vi "UHR-Fleezers Control (host) - 16.2.2v2.vi"() -> ()   [LabVIEW 2014] (continued)
        n2296 = Negate(x=w3289) -> (-x=w3285:dbl)
        n2297 = local write "Scan Range (nm)"(w3285) -> ()
        n2298 = Divide(x=w3311, y=w3339) -> (x/y=w3295:dbl)
        "Scan Increment (MHz)" <- w3295
        n2299 = call "IR AOM freq to word.vi"("Frequency In (MHz)"=w3295) -> ("Frequency Word Out (double)"=w3294:dbl)
        n2300 = Divide(x="Step Size (nm)", y="Scan Speed (nm/s)") -> (x/y=w3282:dbl)
        n2301 = To Quad Integer(1:w3294) -> ()  [unwired: 1 out]
        n2302 = local read "Number Interlace Sets"() -> (w3266:u8)
        n2303 = local read "AI Count (ticks)"() -> (w3267:u16)
        n2304 = local read "Total Counts (ticks)"() -> (w3265:u16)
        n2305 = local read "# Samples/trap"() -> (w3297:u32)
        n2306 = Multiply(x=w3267, y=w3266) -> (x*y=w3264:u16)
        n2307 = Divide(x=w3265, y=w3264) -> (x/y=w3263:dbl)
        n2308 = Select(t=w3298, s="Scan BD", f=w3304) -> (s? t:f=w3336:dbl)
        "Initial freq. (MHz)" <- w3336
        n2309 = Add(x=w3311, y=w3336) -> (x+y=→"Final freq. (MHz)":dbl)
        n2310 = Divide(x=w3265, y=40000000.0) -> (x/y=w3281:dbl)
        n2311 = Divide(x=w3282, y=w3281) -> (x/y=w3280:dbl)
        n2312 = To Unsigned Quad Integer(1:w3280) -> (0:w3255:u64)
        n2313 = Quotient & Remainder(x=w3255, y=u64 2) -> (x-y*floor(x/y)=w3259:u64)  [unwired: 1 out]
        n2314 = Equal?(x=w3259, y=u64 0) -> (x = y?=w3257:bool)
        n2315 = Decrement(x=w3255) -> (x-1=w3256:u64)
        n2316 = Select(t=w3255, s=w3257, f=w3256) -> (s? t:f=w3254:u64)
        "Cycles/step (AOD)" <- w3254
        n2317 = xnode "Read/Write Control"("FPGA VI Reference In"=w3253, "Scan steps"=w3286, "Number of scans"="Number of F/B Scans (AOD)", "Cycles per step"=w3254, "Scan freq.  increment"=w3292, "Scan BD"="Scan BD") -> ("error out"=w3345:errorcluster)  [unwired: 1 in, 1 out]
        n2318 = Multiply(x=w3286, y=w3254) -> (x*y=w3340:u64)
        n2319 = Multiply(x=w3340, y=u64 2) -> (x*y=w3262:u64)
        n2320 = Multiply(x=w3263, y=w3262) -> (x*y=w3261:dbl)
        "Data points/scan (f/b)" <- w3261
        n2321 = Multiply(x=w3261, y="Number of F/B Scans (AOD)") -> (x*y=w3343:dbl)
        "Data points/scans" <- w3343
        n2322 = Divide(x=w3343, y=w3297) -> (x/y=→"N sets should be saved":dbl)
        n2323 = Multiply(x=w3340, y=w3281) -> (x*y=w3279:dbl)
        "Time/Scan (s) (AOD)" <- w3279
        n2324 = Select(t=w3311, s="Scan BD", f=0.0) -> (s? t:f=w3337:dbl)
        n2325 = Select(t=0.0, s="Scan BD", f=w3311) -> (s? t:f=w3333:dbl)
        n2326 = local read "BD 2 Frequency 2 (MHz)"() -> (w3329:dbl)
        n2327 = local read "BD 1 Frequency 2 (MHz)"() -> (w3332:dbl)
        n2328 = Add(x=w3333, y=w3304) -> (x+y=w3330:dbl)
        n2329 = Add(x=w3298, y=w3337) -> (x+y=w3331:dbl)
        n2330 = Multiply(x=w3279, y=2.0) -> (x*y=w3278:dbl)
        n2331 = Multiply(x=w3278, y="Number of F/B Scans (AOD)") -> (x*y=w3275:dbl)
        n2332 = Divide(x=w3275, y=60.0) -> (x/y=→"Time to Finish All (min)":dbl)
        n2333 = Add(x="Trap 2 Bead Size (nm)", y="Trap 1 Bead Size (nm)") -> (x+y=w3319:dbl)
        n2334 = Divide(x=w3319, y=2.0) -> (x/y=w3313:dbl)
        n2335 = local read "Initial delta (MHz)"() -> (w3316:dbl)
        n2336 = Subtract(x=w3330, y=w3329) -> (x-y=w3327:dbl)
        n2337 = Subtract(x=w3331, y=w3332) -> (x-y=w3328:dbl)
        n2338 = Square(x=w3327) -> (x^2=w3326:dbl)
        n2339 = Square(x=w3328) -> (x^2=w3325:dbl)
        n2340 = Add(x=w3325, y=w3326) -> (x+y=w3324:dbl)
        n2341 = Square Root(x=w3324) -> (sqrt(x)=w3323:dbl)
        "Final delta (MHz)" <- w3323
        n2342 = Multiply(x=w3315, y=w3323) -> (x*y=w3322:dbl)
        n2343 = Multiply(x=w3316, y=w3315) -> (x*y=w3314:dbl)
        n2344 = Subtract(x=w3314, y=w3313) -> (x-y=→"Initial sep (nm)":dbl)
        n2345 = Subtract(x=w3322, y=w3313) -> (x-y=→"Final sep (nm)":dbl)
      }
      event "Swap F1 and F2", "RF amplitude switch delay": Value Change {
        n2346 = event-data() -> ()  [unwired: 7 out]
        n2347 = local read "RF amplitude switch delay"() -> (w3347:u16)
        n2348 = local read "Swap F1 and F2"() -> (w3348:bool)
        n2349 = xnode "Read/Write Control"("FPGA VI Reference In"=w3346, "Swap F1 and F2"=w3348, "Amp switch delay"=w3347) -> ("error out"=w3349:errorcluster)  [unwired: 1 in, 1 out]
      }
      event "Scan steps (MCL)", "Number of scans (MCL)", "Scan Range (V)\n(of steps)", "2D or 1D Scan", "N APD Samp/step", "Fast Scan Dir", "Continuous MCL Scanning", "Scan lines (y)": Value Change {
        w3353 = 32767.0 ("y")
        n2350 = event-data() -> ()  [unwired: 7 out]
        n2351 = Select(t="Scan lines (y)", s="2D or 1D Scan", f="Number of scans (MCL)") -> (s? t:f=w3358:u64)
        n2352 = local read "Host fluorescence integration time (s)"() -> (w3350:dbl)
        n2353 = Decrement(x="Scan steps (MCL)") -> (x-1=w3373:u64)
        n2354 = Divide(x="Scan Range (V)\n(of steps)", y=w3373) -> (x/y=w3372:dbl)
        "Desired Scan Incr (V)" <- w3372
        n2355 = Multiply(x=w3372, y=w3353) -> (x*y=w3381:dbl)
        n2356 = Divide(x=w3381, y=10.0) -> (x/y=w3371:dbl)
        "Desired incr (int)" <- w3371
        n2357 = local read "Update Count (MCL)"() -> (w3377:u32)
        n2358 = Round Toward -Infinity(1:w3371) -> (0:w3380:dbl)
        n2359 = To Word Integer(number=w3380) -> (16bit integer=w3356:i16)
        "Actual Incr. int (MCL)" <- w3356
        n2360 = Multiply(x=w3350, y=40000000.0) -> (x*y=w3378:dbl)
        n2361 = Divide(x=w3378, y=w3377) -> (x/y=w3376:dbl)
        n2362 = Multiply(x=i16 10, y=w3356) -> (x*y=w3354:i16)
        n2363 = Multiply(x="N APD Samp/step", y=w3376) -> (x*y=w3375:dbl)
        "Cycles/step (MCL)" <- w3375
        n2364 = Divide(x=w3354, y=w3353) -> (x/y=→"Actual MCL Inc (V)":dbl)
        n2365 = Multiply(x="N APD Samp/step", y="Scan steps (MCL)") -> (x*y=w3367:dbl)
        n2366 = local read "APD Samples/FIFO Acq."() -> (w3365:dbl)
        n2367 = Multiply(x=w3367, y=u64 2) -> (x*y=w3366:dbl)
        "Data points/scan (f+b)" <- w3366
        n2368 = Multiply(x=w3366, y=w3358) -> (x*y=w3384:dbl)
        "Data points/scans (MCL)" <- w3384
        n2369 = Multiply(x=w3350, y=w3366) -> (x*y=w3359:dbl)
        "Time/f+b scan (s) (MCL)" <- w3359
        n2370 = Divide(x=w3384, y=w3365) -> (x/y=→"N sets should be saved (MCL)":dbl)
        n2371 = Multiply(x=w3359, y=w3358) -> (x*y=→"Total Time (s)":dbl)
        n2372 = Not(x="Fast Scan Dir") -> (.not. x?=w3363:bool)
        n2373 = xnode "Read/Write Control"("FPGA VI Reference In"=w3351, "Scan steps (MCL)"="Scan steps (MCL)", "Number of scans (MCL)"=w3358, "Cycles per step (MCL)"=w3375, "Scan freq.  increment (MCL)"=w3356, "1D or 2D Scan?"="2D or 1D Scan", "MCL Scan Axis"=w3363, "Cont. Scan (MCL)"="Continuous MCL Scanning") -> ("error out"=w3386:errorcluster)  [unwired: 1 in, 1 out]
      }
      event "Read Cal": Value Change {
        w3398 = 1000.0 ("y")
        n2374 = event-data() -> ()  [unwired: 7 out]
        n2375 = local read "Save file name"() -> (w3417:path)
        n2376 = local write "Read Cal"(FALSE ("Read Cal")) -> ()
        n2377 = Strip Path(path=w3417) -> (stripped path=w3416:path)  [unwired: 1 out]
        n2378 = Path To String(path=w3416) -> (string=w3415:string)
        n2379 = Concatenate Strings(w3415, "\\current.cal" ("string")) -> (w3413:string)
        n2380 = String To Path(string=w3413) -> (path=w3412:path)
        n2381 = Open/Create/Replace File(file path (use dialog)=w3412, operation (0:open)=T35."open", access (0:read/write)=enum16{"read/write", "read-only", "write-only"}."read-only") -> (refnum out=w3420:refnum<file>, error out=w3406:errorcluster)  [unwired: 1 in, 3 out]
        n2382 = Deny Access(4:w3406, 7:w3420) -> (0:w3405:errorcluster, 3:w3411:refnum<file>)  [unwired: 1 out]
        n2383 = Read from Binary File(5:0.0, 8:w3405, 9:T34."big-endian, network order" ("byte order (0:big-endian, network order)"), 10:-1 ("count (1)"), 11:w3411) -> (0:w3404:errorcluster, 2:w3402:dbl[], 3:w3407:refnum<file>)  [unwired: 2 out]
        n2384 = Array To Cluster(array=w3402) -> (cluster=w3401:T39)
        n2385 = Unbundle(w3401) -> ("[0]"=w3395:dbl, "[1]"=w3389:dbl, "[2]"=w3393:dbl, "[3]"=w3387:dbl, "[4]"=w3400:dbl, "[5]"=w3399:dbl)
        n2386 = Close File(refnum=w3407, error in=w3404) -> (error out=→"Read cal error":errorcluster)  [unwired: 1 out]
        n2387 = Multiply(x=w3400, y=w3398) -> (x*y=w3394:dbl)
        n2388 = Multiply(x=w3399, y=w3398) -> (x*y=w3388:dbl)
        n2389 = Bundle By Name(cluster="T1 calibration", "T1 alpha_x (nm/V)"=w3395, "T1 offset_x (mV)"=w3394, "T1 kappa_x (pN/nm)"=w3393) -> (w3392:T6)
        n2390 = Bundle By Name(cluster="T2 calibration", "T2 alpha_x (nm/V)"=w3389, "T2 offset_x (mV)"=w3388, "T2 kappa_x (pN/nm)"=w3387) -> (w3390:T5)
        n2391 = local write "T1 calibration"(w3392) -> ()
        n2392 = local write "T2 calibration"(w3390) -> ()
      }
      event "Abort MCL Scan": Value Change {
        n2393 = event-data() -> ()  [unwired: 7 out]
        n2394 = local write "MCL Scanning"(FALSE ("MCL Scanning")) -> ()
        n2395 = xnode "Read/Write Control"("FPGA VI Reference In"=w3421, "Abort scan (MCL)"="Abort MCL Scan") -> ("error out"=w3424:errorcluster)  [unwired: 1 in, 1 out]
      }
      event "Update Count (MCL)": Value Change {
        n2396 = event-data() -> ()  [unwired: 7 out]
        n2397 = xnode "Read/Write Control"("FPGA VI Reference In"=w3425, "MCL count"="Update Count (MCL)") -> ("error out"=w3427:errorcluster)  [unwired: 1 in, 1 out]
      }
      event "+ phase (MCL)", "- phase (MCL)": Value Change {
        n2398 = event-data() -> ()  [unwired: 7 out]
        n2399 = Or(x="- phase (MCL)", y="+ phase (MCL)") -> (x .or. y?=w3431:bool)
        n2400 = Negate(x="Phase adjust (MCL)") -> (-x=w3437:i16)
        n2401 = Select(t=w3437, s="+ phase (MCL)", f="Phase adjust (MCL)") -> (s? t:f=w3435:i16)
        n2402 = xnode "Read/Write Control"("FPGA VI Reference In"=w3428, "Phase count adjustment (MCL)"=w3435) -> ("FPGA VI Reference Out"=w3432:T25, "error out"=w3433:errorcluster)  [unwired: 1 in]
        n2403 = xnode "Read/Write Control"("FPGA VI Reference In"=w3432, "error in"=w3433, "+ phase (MCL)"=w3431) -> ("error out"=w3430:errorcluster)  [unwired: 1 out]
      }
      event "Abort AOD Scan": Value Change {
        n2404 = event-data() -> ()  [unwired: 7 out]
        n2405 = xnode "Read/Write Control"("FPGA VI Reference In"=w3438, "Abort scan"="Abort AOD Scan") -> ("error out"=w3440:errorcluster)  [unwired: 1 in, 1 out]
      }
      event "Continuous AOD Scanning": Value Change {
        n2406 = event-data() -> ()  [unwired: 7 out]
        n2407 = xnode "Read/Write Control"("FPGA VI Reference In"=w3441, "Cont. Scan"="Continuous AOD Scanning") -> ("error out"=w3443:errorcluster)  [unwired: 1 in, 1 out]
      }
      event "Index": Value Change {
        n2408 = event-data() -> ()  [unwired: 7 out]
        n2409 = call "Create new save file.vi"("Insert"="", "Ext"=".dat" ("string"), "Index In"="Index") -> ("Path Out"=→"Save file name":path, "Index Out"=w3444:dbl)
        "Save index" <- w3444
        n2410 = local write "Index"(w3444) -> ()
      }
      event "AO1", "AO2": Value Change {
        w3458 = 10.0 ("y")
        w3457 = 32767.0 ("y")
        n2411 = event-data() -> ()  [unwired: 7 out]
        n2412 = local read "AO2"() -> (w3456:dbl)
        n2413 = local read "AO1"() -> (w3453:dbl)
        n2414 = Multiply(x=w3453, y=w3457) -> (x*y=w3452:dbl)
        n2415 = Multiply(x=w3456, y=w3457) -> (x*y=w3455:dbl)
        n2416 = Divide(x=w3452, y=w3458) -> (x/y=w3451:dbl)
        n2417 = Divide(x=w3455, y=w3458) -> (x/y=w3454:dbl)
        n2418 = To Word Integer(number=w3451) -> (16bit integer=w3459:i16)
        n2419 = To Word Integer(number=w3454) -> (16bit integer=w3460:i16)
        n2420 = xnode "Read/Write Control"("FPGA VI Reference In"=w3449, "AO1"=w3459, "AO2"=w3460) -> ("error out"=w3450:errorcluster)  [unwired: 1 in, 1 out]
      }
      event "Inject Pump 1": Value Change {
        n2421 = event-data() -> ()  [unwired: 7 out]
        n2422 = local read "Use Harvard pumps\nfor beads (else Chemyx)"() -> (w3462:bool)
        n2423 = case shown="True" w3462 {
          tunnel: "Inject Pump 1" -> [w3466 w3507]
          tunnel: w3461 -> [_ w3508]
          frame False {
            n2424 = local read "Pump write delay (ms)"() -> (w3465:dbl)
            n2425 = local read "Chemyx Syringe Pump Serial Port"() -> (w3464:refnum<visa-resource-name>)
            n2426 = case shown="True" w3466 {
              tunnel: w3465 -> [w3472 w3486]
              tunnel: w3464 -> [w3469 w3485]
              frame False {
                n2427 = flat-sequence {
                  tunnel: w3469 -> [w3473]
                  tunnel: [w3473] -> w3470
                  tunnel: w3472 -> [_]
                  tunnel: [w3476] -> w3471
                  tunnel: w3470 -> [w3476]
                  tunnel: w3471 -> [w3477]
                  tunnel: [w3477] -> w3467
                  tunnel: [w3479] -> w3468
                  tunnel: w3467 -> [w3479]
                  tunnel: w3468 -> [w3481]
                  frame #0 {
                    n2428 = call "Write to pump.vi"("string"="enter pump1", "VISA resource name"=w3473) -> ()  [unwired: 1 out]
                  }
                  frame #1 {
                    n2429 = Wait (ms)(milliseconds to wait="Pump pause delay (ms)") -> ()  [unwired: 1 out]
                  }
                  frame #2 {
                    n2430 = call "Write to pump.vi"("string"="stop", "VISA resource name"=w3477) -> ()  [unwired: 1 out]
                  }
                  frame #3 {
                    n2431 = Wait (ms)(milliseconds to wait=u32 500) -> ()  [unwired: 1 out]
                  }
                  frame #4 {
                    n2432 = call "Write to pump.vi"("string"="stop", "VISA resource name"=w3481) -> ()  [unwired: 1 out]
                  }
                }
              }
              frame True {
                n2433 = flat-sequence {
                  tunnel: w3485 -> [w3495]
                  tunnel: w3486 -> [w3490]
                  tunnel: w3486 -> [w3497]
                  tunnel: w3485 -> [w3498]
                  tunnel: [w3498] -> w3483
                  tunnel: [w3500] -> w3484
                  tunnel: w3483 -> [w3500]
                  tunnel: w3484 -> [w3502]
                  frame #0 {
                    n2434 = local read "All Pump Parameters"() -> (w3489:T7)
                    n2435 = Unbundle By Name(w3489) -> ("Pump 1"=w3496:T40)
                    n2436 = call "Set pump parameters.vi"("Pump write delay (ms)"=w3490, "Volume (uL)"="Ch 1 Inject Volume (uL)", "Rate (uL/h)"="Ch 1 Inject Rate (ul/h)", "Units"=4.0, "Pump #"=1.0, "Pump Parameters In"=w3496, "VISA resource name"=w3495) -> ("Pump Parameters Out"=w3488:T40)  [unwired: 3 in]
                    n2437 = Bundle By Name(cluster=w3489, "Pump 1"=w3488) -> (w3487:T7)
                    n2438 = local write "All Pump Parameters"(w3487) -> ()
                  }
                  frame #1 {
                    n2439 = Wait (ms)(milliseconds to wait=w3497) -> ()  [unwired: 1 out]
                  }
                  frame #2 {
                    n2440 = call "Write to pump.vi"("string"="start", "VISA resource name"=w3498) -> ()  [unwired: 1 out]
                  }
                  frame #3 {
                    n2441 = Wait (ms)(milliseconds to wait=u32 500) -> ()  [unwired: 1 out]
                  }
                  frame #4 {
                    n2442 = call "Write to pump.vi"("string"="start", "VISA resource name"=w3502) -> ()  [unwired: 1 out]
                  }
                }
              }
            }
          }
          frame True {
            n2443 = case shown="False" w3507 {
              tunnel: w3508 -> [w3520 w3530]
              frame False {
                n2444 = flat-sequence {
                  tunnel: w3520 -> [w3522]
                  frame #0 {
                    n2445 = local write "Flushing P1"(FALSE ("Flushing P1")) -> ()
                    n2446 = Concatenate Strings("stop" ("string"), "\r") -> (w3524:string)
                    n2447 = VISA Write(VISA resource name=w3522, write buffer=w3524) -> ()  [unwired: 1 in, 3 out]
                  }
                  frame #1 {
                    n2448 = property on="Clear Volume P1" class="Bool (strict)"("Val(Sgnl)"=TRUE ("Value (Signaling)")) -> ()  [unwired: 2 in, 2 out]
                  }
                }
              }
              frame True {
                n2449 = local read "Normal Flow Rate (ul/h) P1"() -> (w3528:dbl)
                n2450 = Number To Decimal String(number=w3528) -> (decimal integer string=w3534:string)  [unwired: 1 in]
                n2451 = Concatenate Strings("irate  " ("string"), w3534, " u/h" ("string"), "\r") -> (w3532:string)
                n2452 = VISA Write(VISA resource name=w3530, write buffer=w3532) -> (VISA resource name out=w3529:refnum<visa-resource-name>)  [unwired: 1 in, 2 out]
                n2453 = Concatenate Strings("irun" ("string"), "\r") -> (w3536:string)
                n2454 = VISA Write(VISA resource name=w3529, write buffer=w3536) -> ()  [unwired: 1 in, 3 out]
              }
            }
            n2455 = local read "Saving..."() -> (w3505:bool)
            n2456 = local read "Save Event Log?"() -> (w3504:bool)
            n2457 = And(x=w3505, y=w3504) -> (x .and. y?=w3506:bool)
            n2458 = case shown="True" w3506 {
              tunnel: w3507 -> [_ w3518]
              frame False {
              }
              frame True {
                n2459 = local read "Normal Flow Rate (ul/h) P1"() -> (w3509:dbl)
                n2460 = Number To Decimal String(number=w3509) -> (decimal integer string=w3510:string)  [unwired: 1 in]
                n2461 = Concatenate Strings("on, flow rate", w3510) -> (w3512:string)
                n2462 = Select(t=w3512, s=w3518, f="off") -> (s? t:f=w3514:string)
                n2463 = local read "log file ref"() -> (w3519:refnum<file>)
                n2464 = local read "Time (s)"() -> (w3513:dbl)
                n2465 = Concatenate Strings("pump 1 ", w3514) -> (w3516:string)
                n2466 = call "write to event log.vi"("log file ref"=w3519, "time"=w3513, "input string"=w3516) -> ()  [unwired: 8 in]
              }
            }
          }
        }
      }
      event "Inject Pump 3": Value Change {
        n2467 = event-data() -> ()  [unwired: 7 out]
        n2468 = local read "Use Harvard pumps\nfor beads (else Chemyx)"() -> (w3539:bool)
        n2469 = case shown="True" w3539 {
          tunnel: "Inject Pump 3" -> [w3543 w3584]
          tunnel: w3538 -> [_ w3585]
          frame False {
            n2470 = local read "Pump write delay (ms)"() -> (w3542:dbl)
            n2471 = case shown="True" w3543 {
              tunnel: w3542 -> [w3549 w3563]
              tunnel: "Chemyx Syringe Pump Serial Port" -> [w3546 w3562]
              frame False {
                n2472 = flat-sequence {
                  tunnel: w3546 -> [w3550]
                  tunnel: [w3550] -> w3547
                  tunnel: w3549 -> [_]
                  tunnel: [w3553] -> w3548
                  tunnel: w3547 -> [w3553]
                  tunnel: w3548 -> [w3554]
                  tunnel: [w3554] -> w3544
                  tunnel: [w3556] -> w3545
                  tunnel: w3544 -> [w3556]
                  tunnel: w3545 -> [w3558]
                  frame #0 {
                    n2473 = call "Write to pump.vi"("string"="enter pump3", "VISA resource name"=w3550) -> ()  [unwired: 1 out]
                  }
                  frame #1 {
                    n2474 = local read "Pump pause delay (ms)"() -> (w3552:u32)
                    n2475 = Wait (ms)(milliseconds to wait=w3552) -> ()  [unwired: 1 out]
                  }
                  frame #2 {
                    n2476 = call "Write to pump.vi"("string"="stop", "VISA resource name"=w3554) -> ()  [unwired: 1 out]
                  }
                  frame #3 {
                    n2477 = Wait (ms)(milliseconds to wait=u32 0) -> ()  [unwired: 1 out]
                  }
                  frame #4 {
                    n2478 = call "Write to pump.vi"("string"="stop", "VISA resource name"=w3558) -> ()  [unwired: 1 out]
                  }
                }
              }
              frame True {
                n2479 = flat-sequence {
                  tunnel: w3562 -> [w3572]
                  tunnel: w3563 -> [w3567]
                  tunnel: w3563 -> [w3574]
                  tunnel: w3562 -> [w3575]
                  tunnel: [w3575] -> w3561
                  tunnel: [w3578] -> w3560
                  tunnel: w3561 -> [w3578]
                  tunnel: w3560 -> [w3579]
                  frame #0 {
                    n2480 = local read "All Pump Parameters"() -> (w3566:T7)
                    n2481 = Unbundle By Name(w3566) -> ("Pump 3"=w3573:T40)
                    n2482 = call "Set pump parameters.vi"("Pump write delay (ms)"=w3567, "Volume (uL)"="Ch 3 Inject Volume (uL)", "Rate (uL/h)"="Ch 3 Inject Rate (ul/h)", "Units"=4.0, "Pump #"=3.0, "Pump Parameters In"=w3573, "VISA resource name"=w3572) -> ("Pump Parameters Out"=w3565:T40)  [unwired: 3 in]
                    n2483 = Bundle By Name(cluster=w3566, "Pump 3"=w3565) -> (w3564:T7)
                    n2484 = local write "All Pump Parameters"(w3564) -> ()
                  }
                  frame #1 {
                    n2485 = Wait (ms)(milliseconds to wait=w3574) -> ()  [unwired: 1 out]
                  }
                  frame #2 {
                    n2486 = call "Write to pump.vi"("string"="start", "VISA resource name"=w3575) -> ()  [unwired: 1 out]
                  }
                  frame #3 {
                    n2487 = Wait (ms)(milliseconds to wait=u32 500) -> ()  [unwired: 1 out]
                  }
                  frame #4 {
                    n2488 = call "Write to pump.vi"("string"="start", "VISA resource name"=w3579) -> ()  [unwired: 1 out]
                  }
                }
              }
            }
          }
          frame True {
            n2489 = case shown="False" w3584 {
              tunnel: w3585 -> [w3597 w3604]
              frame False {
                n2490 = flat-sequence {
                  tunnel: w3597 -> [w3599]
                  frame #0 {
                    n2491 = local write "Flushing P3"(FALSE ("Flushing P3")) -> ()
                    n2492 = Concatenate Strings("stop" ("string"), "\r") -> (w3601:string)
                    n2493 = VISA Write(VISA resource name=w3599, write buffer=w3601) -> ()  [unwired: 1 in, 3 out]
                  }
                  frame #1 {
                    n2494 = property on="Clear Volume P3" class="Bool (strict)"("Val(Sgnl)"=TRUE ("Value (Signaling)")) -> ()  [unwired: 2 in, 2 out]
                  }
                }
              }
              frame True {
                n2495 = local read "Normal Flow Rate (ul/h) P3"() -> (w3605:dbl)
                n2496 = Number To Decimal String(number=w3605) -> (decimal integer string=w3611:string)  [unwired: 1 in]
                n2497 = Concatenate Strings("irate  " ("string"), w3611, " u/h" ("string"), "\r") -> (w3609:string)
                n2498 = VISA Write(VISA resource name=w3604, write buffer=w3609) -> (VISA resource name out=w3607:refnum<visa-resource-name>)  [unwired: 1 in, 2 out]
                n2499 = Concatenate Strings("irun" ("string"), "\r") -> (w3613:string)
                n2500 = VISA Write(VISA resource name=w3607, write buffer=w3613) -> ()  [unwired: 1 in, 3 out]
              }
            }
            n2501 = local read "Save Event Log?"() -> (w3582:bool)
            n2502 = local read "Saving..."() -> (w3583:bool)
            n2503 = And(x=w3583, y=w3582) -> (x .and. y?=w3581:bool)
            n2504 = case shown="True" w3581 {
              tunnel: w3584 -> [_ w3592]
              frame False {
              }
              frame True {
                n2505 = local read "Normal Flow Rate (ul/h) P3"() -> (w3586:dbl)
                n2506 = Number To Decimal String(number=w3586) -> (decimal integer string=w3588:string)  [unwired: 1 in]
                n2507 = Concatenate Strings("on, flow rate", w3588) -> (w3587:string)
                n2508 = local read "log file ref"() -> (w3591:refnum<file>)
                n2509 = Select(t=w3587, s=w3592, f="off") -> (s? t:f=w3593:string)
                n2510 = local read "Time (s)"() -> (w3590:dbl)
                n2511 = Concatenate Strings("pump 3 ", w3593) -> (w3595:string)
                n2512 = call "write to event log.vi"("log file ref"=w3591, "time"=w3590, "input string"=w3595) -> ()  [unwired: 8 in]
              }
            }
          }
        }
      }
      event "Inject Pump 2": Value Change {
        n2513 = event-data() -> ()  [unwired: 7 out]
        n2514 = local read "Pump write delay (ms)"() -> (w3620:dbl)
        n2515 = flat-sequence {
          tunnel: w3619 -> [w3644]
          tunnel: w3620 -> [w3640]
          tunnel: "Inject Pump 2" -> [_]
          tunnel: w3620 -> [w3646]
          tunnel: w3619 -> [w3647]
          frame #0 {
            n2516 = local read "All Pump Parameters"() -> (w3639:T7)
            n2517 = Multiply(x=60.0, y="Flush Center Ch Rate (ul/m)") -> (x*y=w3636:dbl)
            n2518 = Unbundle By Name(w3639) -> ("Pump 2"=w3645:T40)
            n2519 = call "Set pump parameters.vi"("Pump write delay (ms)"=w3640, "Volume (uL)"="Flush Center Ch Volume (uL)", "Rate (uL/h)"=w3636, "Units"=3.0, "Pump #"=2.0, "Pump Parameters In"=w3645, "VISA resource name"=w3644) -> ("Pump Parameters Out"=w3638:T40)  [unwired: 3 in]
            n2520 = Bundle By Name(cluster=w3639, "Pump 2"=w3638) -> (w3637:T7)
            n2521 = local write "All Pump Parameters"(w3637) -> ()
            n2522 = Add(x="Flush Center Ch Volume (uL)", y="Total Volume\nFlushed (uL)") -> (x+y=w3633:dbl)
            n2523 = local write "Total Volume\nFlushed (uL)"(w3633) -> ()
          }
          frame #1 {
            n2524 = Wait (ms)(milliseconds to wait=w3646) -> ()  [unwired: 1 out]
          }
          frame #2 {
            n2525 = call "Write to pump.vi"("string"="start", "VISA resource name"=w3647) -> ()  [unwired: 1 out]
          }
        }
        n2526 = local read "Chemyx Syringe Pump Serial Port"() -> (w3619:refnum<visa-resource-name>)
        n2527 = local read "Save Event Log?"() -> (w3618:bool)
        n2528 = local read "Saving..."() -> (w3617:bool)
        n2529 = And(x=w3618, y=w3617) -> (x .and. y?=w3616:bool)
        n2530 = case shown="True" w3616 {
          tunnel: "Inject Pump 2" -> [_ w3627]
          frame False {
          }
          frame True {
            n2531 = local read "Flow rate (uL/h)"() -> (w3621:dbl)
            n2532 = Number To Decimal String(number=w3621) -> (decimal integer string=w3623:string)  [unwired: 1 in]
            n2533 = Concatenate Strings("on, flow rate", w3623) -> (w3622:string)
            n2534 = Select(t=w3622, s=w3627, f="off") -> (s? t:f=w3631:string)
            n2535 = local read "Time (s)"() -> (w3625:dbl)
            n2536 = local read "log file ref"() -> (w3626:refnum<file>)
            n2537 = Concatenate Strings("pump 2 ", w3631) -> (w3629:string)
            n2538 = call "write to event log.vi"("log file ref"=w3626, "time"=w3625, "input string"=w3629) -> ()  [unwired: 8 in]
          }
        }
      }
      event "Sample Channel\nFlow": Value Change {
        n2539 = event-data() -> ()  [unwired: 7 out]
        n2540 = Select(t="irun" ("string"), s="Sample Channel\nFlow", f="stop" ("string")) -> (s? t:f=w3651:string)
        n2541 = Concatenate Strings(w3651, "\r") -> (w3654:string)
        n2542 = VISA Write(VISA resource name=w3649, write buffer=w3654) -> ()  [unwired: 1 in, 3 out]
      }
      event "Start Flow": Value Change {
        n2543 = event-data() -> ()  [unwired: 7 out]
        n2544 = local write "Sample Channel\nFlow"(TRUE ("Sample Channel\nFlow")) -> ()
        n2545 = local write "Start Flow"(FALSE ("Start Flow")) -> ()
        n2546 = Concatenate Strings("irun" ("string"), "\r") -> (w3660:string)
        n2547 = VISA Write(VISA resource name=w3656, write buffer=w3660) -> ()  [unwired: 1 in, 3 out]
      }
      event "Stop Flow": Value Change {
        w3662 = FALSE ("Stop Flow")
        n2548 = event-data() -> ()  [unwired: 7 out]
        n2549 = local write "Stop Flow"(w3662) -> ()
        n2550 = local write "Sample Channel\nFlow"(w3662) -> ()
        n2551 = Concatenate Strings("stop" ("string"), "\r") -> (w3665:string)
        n2552 = VISA Write(VISA resource name=w3663, write buffer=w3665) -> ()  [unwired: 1 in, 3 out]
      }
      event "Flow rate (uL/h)": Value Change {
        n2553 = event-data() -> ()  [unwired: 7 out]
        n2554 = Number To Decimal String(number="Flow rate (uL/h)") -> (decimal integer string=w3672:string)  [unwired: 1 in]
        n2555 = Concatenate Strings("irate  " ("string"), w3672, " u/h" ("string"), "\r") -> (w3671:string)
        n2556 = VISA Write(VISA resource name=w3668, write buffer=w3671) -> ()  [unwired: 1 in, 3 out]
      }
      event "Flush Sample": Value Change {
        n2557 = event-data() -> ()  [unwired: 7 out]
        n2558 = flat-sequence {
          tunnel: w3682 -> [w3720]
          tunnel: [w3700] -> w3681
          tunnel: [w3696] -> w3679
          tunnel: ["Volume (uL)"] -> w3678
          tunnel: ["Flush rate (uL/m)"] -> w3677
          tunnel: w3681 -> [w3724]
          tunnel: [w3724] -> w3680
          tunnel: w3679 -> [w3723]
          tunnel: w3680 -> [w3729]
          frame #0 {
            # "set paramaters (rate, volume) for flush, clear volume"
            n2559 = Number To Decimal String(number="Flush rate (uL/m)") -> (decimal integer string=w3716:string)  [unwired: 1 in]
            n2560 = Concatenate Strings("irate  " ("string"), w3716, " u/m" ("string"), "\r") -> (w3718:string)
            n2561 = VISA Write(VISA resource name=w3720, write buffer=w3718) -> (VISA resource name out=w3714:refnum<visa-resource-name>)  [unwired: 1 in, 2 out]
            n2562 = Reciprocal(x="Flush rate (uL/m)") -> (1/x=w3699:dbl)
            n2563 = Number To Decimal String(number="Volume (uL)") -> (decimal integer string=w3705:string)  [unwired: 1 in]
            n2564 = Multiply(x="Volume (uL)", y=w3699) -> (x*y=w3698:dbl)
            n2565 = Concatenate Strings("tvolume  " ("string"), w3705, " u" ("string"), "\r") -> (w3703:string)
            n2566 = Multiply(x=w3698, y=60000.0) -> (x*y=w3696:dbl)
            n2567 = VISA Write(VISA resource name=w3714, write buffer=w3703) -> (VISA resource name out=w3702:refnum<visa-resource-name>)  [unwired: 1 in, 2 out]
            n2568 = Concatenate Strings("cvolume" ("string"), "\r") -> (w3701:string)
            n2569 = VISA Write(VISA resource name=w3702, write buffer=w3701) -> (VISA resource name out=w3712:refnum<visa-resource-name>)  [unwired: 1 in, 2 out]
            n2570 = Concatenate Strings("irun" ("string"), "\r") -> (w3710:string)
            n2571 = VISA Write(VISA resource name=w3712, write buffer=w3710) -> (VISA resource name out=w3700:refnum<visa-resource-name>)  [unwired: 1 in, 2 out]
          }
          frame #1 {
            # "Have to wait until\nflow is done to reset\nrate"
            n2572 = Add(x=w3723, y=100.0) -> (x+y=w3722:dbl)
            n2573 = Wait (ms)(milliseconds to wait=w3722) -> ()  [unwired: 1 out]
          }
          frame #2 {
            # "reset flow rate to usual flow rate"
            n2574 = local read "Flow rate (uL/h)"() -> (w3735:dbl)
            n2575 = Number To Decimal String(number=w3735) -> (decimal integer string=w3733:string)  [unwired: 1 in]
            n2576 = Concatenate Strings("irate  " ("string"), w3733, " u/h" ("string"), "\r") -> (w3731:string)
            n2577 = VISA Write(VISA resource name=w3729, write buffer=w3731) -> (VISA resource name out=w3725:refnum<visa-resource-name>)  [unwired: 1 in, 2 out]
            n2578 = Concatenate Strings("cvolume" ("string"), "\r") -> (w3726:string)
            n2579 = VISA Write(VISA resource name=w3725, write buffer=w3726) -> ()  [unwired: 1 in, 3 out]
          }
        }
        n2580 = local read "Save Event Log?"() -> (w3675:bool)
        n2581 = local read "Saving..."() -> (w3674:bool)
        n2582 = And(x=w3675, y=w3674) -> (x .and. y?=w3676:bool)
        n2583 = case shown="True" w3676 {
          tunnel: w3678 -> [_ w3685]
          tunnel: w3677 -> [_ w3684]
          frame False {
          }
          frame True {
            n2584 = Number To Decimal String(number=w3685) -> (decimal integer string=w3689:string)  [unwired: 1 in]
            n2585 = Number To Decimal String(number=w3684) -> (decimal integer string=w3691:string)  [unwired: 1 in]
            n2586 = local read "log file ref"() -> (w3686:refnum<file>)
            n2587 = local read "Time (s)"() -> (w3687:dbl)
            n2588 = Concatenate Strings("pump 2 flushing ", w3689, " uL at ", w3691, " ul/min") -> (w3693:string)
            n2589 = call "write to event log.vi"("log file ref"=w3686, "time"=w3687, "input string"=w3693) -> ()  [unwired: 8 in]
          }
        }
      }
      event "Flush Pump 3": Value Change {
        n2590 = event-data() -> ()  [unwired: 7 out]
        n2591 = flat-sequence {
          tunnel: w3741 -> [w3756]
          tunnel: ["Flush rate (uL/m) P3"] -> w3737
          tunnel: ["Volume (uL) P3"] -> w3736
          frame #0 {
            # "set paramaters (rate, volume) for flush, clear volume"
            n2592 = Number To Decimal String(number="Flush rate (uL/m) P3") -> (decimal integer string=w3776:string)  [unwired: 1 in]
            n2593 = local write "Inject Pump 3"(TRUE ("Inject Pump 3")) -> ()
            n2594 = Concatenate Strings("irate  " ("string"), w3776, " u/m" ("string"), "\r") -> (w3778:string)
            n2595 = VISA Write(VISA resource name=w3756, write buffer=w3778) -> (VISA resource name out=w3774:refnum<visa-resource-name>)  [unwired: 1 in, 2 out]
            n2596 = Reciprocal(x="Flush rate (uL/m) P3") -> (1/x=w3760:dbl)
            n2597 = Number To Decimal String(number="Volume (uL) P3") -> (decimal integer string=w3765:string)  [unwired: 1 in]
            n2598 = Multiply(x="Volume (uL) P3", y=w3760) -> (x*y=w3759:dbl)
            n2599 = Concatenate Strings("tvolume  " ("string"), w3765, " u" ("string"), "\r") -> (w3763:string)
            n2600 = Multiply(x=w3759, y=60.0) -> (x*y=→"HP3 Flush Time (s)":dbl)
            n2601 = VISA Write(VISA resource name=w3774, write buffer=w3763) -> (VISA resource name out=w3762:refnum<visa-resource-name>)  [unwired: 1 in, 2 out]
            n2602 = Concatenate Strings("cvolume" ("string"), "\r") -> (w3761:string)
            n2603 = VISA Write(VISA resource name=w3762, write buffer=w3761) -> (VISA resource name out=w3772:refnum<visa-resource-name>)  [unwired: 1 in, 2 out]
            n2604 = Concatenate Strings("irun" ("string"), "\r") -> (w3770:string)
            n2605 = VISA Write(VISA resource name=w3772, write buffer=w3770) -> ()  [unwired: 1 in, 3 out]
          }
          frame #1 {
            "Flushing P3" <- TRUE ("Flushing P3")
          }
        }
        n2606 = local read "Save Event Log?"() -> (w3739:bool)
        n2607 = local read "Saving..."() -> (w3740:bool)
        n2608 = And(x=w3739, y=w3740) -> (x .and. y?=w3738:bool)
        n2609 = case shown="True" w3738 {
          tunnel: w3737 -> [_ w3744]
          tunnel: w3736 -> [_ w3743]
          frame False {
          }
          frame True {
            n2610 = Number To Decimal String(number=w3743) -> (decimal integer string=w3748:string)  [unwired: 1 in]
            n2611 = Number To Decimal String(number=w3744) -> (decimal integer string=w3750:string)  [unwired: 1 in]
            n2612 = local read "log file ref"() -> (w3745:refnum<file>)
            n2613 = local read "Time (s)"() -> (w3746:dbl)
            n2614 = Concatenate Strings("pump 3 flushing ", w3748, " uL at ", w3750, " ul/min") -> (w3752:string)
            n2615 = call "write to event log.vi"("log file ref"=w3745, "time"=w3746, "input string"=w3752) -> ()  [unwired: 8 in]
          }
        }
      }
      event "Flush Pump 1": Value Change {
        n2616 = event-data() -> ()  [unwired: 7 out]
        n2617 = flat-sequence {
          tunnel: [w3807] -> w3787
          tunnel: w3786 -> [w3802]
          tunnel: ["Volume (uL) P1"] -> w3782
          tunnel: ["Flush rate (uL/m) P1"] -> w3781
          tunnel: w3787 -> [_]
          frame #0 {
            # "set paramaters (rate, volume) for flush, clear volume"
            n2618 = local write "Inject Pump 1"(TRUE ("Inject Pump 1")) -> ()
            n2619 = Number To Decimal String(number="Flush rate (uL/m) P1") -> (decimal integer string=w3823:string)  [unwired: 1 in]
            n2620 = Concatenate Strings("irate  " ("string"), w3823, " u/m" ("string"), "\r") -> (w3825:string)
            n2621 = VISA Write(VISA resource name=w3802, write buffer=w3825) -> (VISA resource name out=w3821:refnum<visa-resource-name>)  [unwired: 1 in, 2 out]
            n2622 = Reciprocal(x="Flush rate (uL/m) P1") -> (1/x=w3806:dbl)
            n2623 = Number To Decimal String(number="Volume (uL) P1") -> (decimal integer string=w3812:string)  [unwired: 1 in]
            n2624 = Multiply(x="Volume (uL) P1", y=w3806) -> (x*y=w3805:dbl)
            n2625 = Concatenate Strings("tvolume  " ("string"), w3812, " u" ("string"), "\r") -> (w3810:string)
            n2626 = Multiply(x=w3805, y=60.0) -> (x*y=→"HP1 Flush Time (s)":dbl)
            n2627 = VISA Write(VISA resource name=w3821, write buffer=w3810) -> (VISA resource name out=w3809:refnum<visa-resource-name>)  [unwired: 1 in, 2 out]
            n2628 = Concatenate Strings("cvolume" ("string"), "\r") -> (w3808:string)
            n2629 = VISA Write(VISA resource name=w3809, write buffer=w3808) -> (VISA resource name out=w3819:refnum<visa-resource-name>)  [unwired: 1 in, 2 out]
            n2630 = Concatenate Strings("irun" ("string"), "\r") -> (w3817:string)
            n2631 = VISA Write(VISA resource name=w3819, write buffer=w3817) -> (VISA resource name out=w3807:refnum<visa-resource-name>)  [unwired: 1 in, 2 out]
          }
          frame #1 {
            "Flushing P1" <- TRUE ("Flushing P3")
          }
        }
        n2632 = local read "Saving..."() -> (w3783:bool)
        n2633 = local read "Save Event Log?"() -> (w3784:bool)
        n2634 = And(x=w3784, y=w3783) -> (x .and. y?=w3785:bool)
        n2635 = case shown="True" w3785 {
          tunnel: w3782 -> [_ w3791]
          tunnel: w3781 -> [_ w3790]
          frame False {
          }
          frame True {
            n2636 = Number To Decimal String(number=w3791) -> (decimal integer string=w3795:string)  [unwired: 1 in]
            n2637 = Number To Decimal String(number=w3790) -> (decimal integer string=w3793:string)  [unwired: 1 in]
            n2638 = local read "log file ref"() -> (w3797:refnum<file>)
            n2639 = local read "Time (s)"() -> (w3798:dbl)
            n2640 = Concatenate Strings("pump 1 flushing ", w3795, " uL at ", w3793, " ul/min") -> (w3789:string)
            n2641 = call "write to event log.vi"("log file ref"=w3797, "time"=w3798, "input string"=w3789) -> ()  [unwired: 8 in]
          }
        }
      }
      event "Clear Volume": Value Change {
        n2642 = event-data() -> ()  [unwired: 7 out]
        n2643 = Concatenate Strings("cvolume" ("string"), "\r") -> (w3829:string)
        n2644 = VISA Write(VISA resource name=w3828, write buffer=w3829) -> ()  [unwired: 1 in, 3 out]
      }
      event "Clear Volume P3": Value Change {
        n2645 = event-data() -> ()  [unwired: 7 out]
        n2646 = Concatenate Strings("cvolume" ("string"), "\r") -> (w3835:string)
        n2647 = VISA Write(VISA resource name=w3834, write buffer=w3835) -> ()  [unwired: 1 in, 3 out]
        n2648 = local write "Clear Volume P3"(FALSE ("Clear Volume P3")) -> ()
      }
      event "Clear Volume P1": Value Change {
        n2649 = event-data() -> ()  [unwired: 7 out]
        n2650 = Concatenate Strings("cvolume" ("string"), "\r") -> (w3840:string)
        n2651 = local write "Clear Volume P1"(FALSE ("Clear Volume P1")) -> ()
        n2652 = VISA Write(VISA resource name=w3839, write buffer=w3840) -> ()  [unwired: 1 in, 3 out]
      }
      event "Display On P3": Value Change {
        n2653 = event-data() -> ()  [unwired: 7 out]
        n2654 = Select(t="dim 100", s="Display On P3", f="dim 0") -> (s? t:f=w3846:string)
        n2655 = Concatenate Strings(w3846, "\r") -> (w3848:string)
        n2656 = VISA Write(VISA resource name=w3843, write buffer=w3848) -> ()  [unwired: 1 in, 3 out]
      }
      event "Display On P1": Value Change {
        n2657 = event-data() -> ()  [unwired: 7 out]
        n2658 = Select(t="dim 100", s="Display On P1", f="dim 0") -> (s? t:f=w3853:string)
        n2659 = Concatenate Strings(w3853, "\r") -> (w3855:string)
        n2660 = VISA Write(VISA resource name=w3850, write buffer=w3855) -> ()  [unwired: 1 in, 3 out]
      }
      event "Retract Pump 3": Value Change {
        n2661 = event-data() -> ()  [unwired: 7 out]
        n2662 = local write "Retract Pump 3"(FALSE ("Retract Pump 3")) -> ()
        n2663 = case shown="True" "Retract Pump 3" {
          tunnel: w3857 -> [_ w3860]
          frame False {
          }
          frame True {
            n2664 = Number To Decimal String(number="Retract Rate (uL/m)") -> (decimal integer string=w3878:string)  [unwired: 1 in]
            n2665 = Concatenate Strings("wrate  " ("string"), w3878, " u/m" ("string"), "\r") -> (w3880:string)
            n2666 = VISA Write(VISA resource name=w3860, write buffer=w3880) -> (VISA resource name out=w3871:refnum<visa-resource-name>)  [unwired: 1 in, 2 out]
            n2667 = Number To Decimal String(number="Retract Vol 3 (uL)") -> (decimal integer string=w3873:string)  [unwired: 1 in]
            n2668 = Concatenate Strings("tvolume  " ("string"), w3873, " u" ("string"), "\r") -> (w3870:string)
            n2669 = VISA Write(VISA resource name=w3871, write buffer=w3870) -> (VISA resource name out=w3866:refnum<visa-resource-name>)  [unwired: 1 in, 2 out]
            n2670 = Concatenate Strings("cvolume" ("string"), "\r") -> (w3867:string)
            n2671 = VISA Write(VISA resource name=w3866, write buffer=w3867) -> (VISA resource name out=w3861:refnum<visa-resource-name>)  [unwired: 1 in, 2 out]
            n2672 = Concatenate Strings("wrun" ("string"), "\r") -> (w3862:string)
            n2673 = VISA Write(VISA resource name=w3861, write buffer=w3862) -> ()  [unwired: 1 in, 3 out]
          }
        }
      }
      event "Retract Pump 1": Value Change {
        n2674 = event-data() -> ()  [unwired: 7 out]
        n2675 = local write "Retract Pump 1"(FALSE ("Retract Pump 1")) -> ()
        n2676 = case shown="True" "Retract Pump 1" {
          tunnel: w3882 -> [_ w3887]
          frame False {
          }
          frame True {
            n2677 = local read "Retract Rate (uL/m)"() -> (w3885:dbl)
            n2678 = Number To Decimal String(number=w3885) -> (decimal integer string=w3903:string)  [unwired: 1 in]
            n2679 = Concatenate Strings("wrate  " ("string"), w3903, " u/m" ("string"), "\r") -> (w3905:string)
            n2680 = VISA Write(VISA resource name=w3887, write buffer=w3905) -> (VISA resource name out=w3897:refnum<visa-resource-name>)  [unwired: 1 in, 2 out]
            n2681 = Number To Decimal String(number="Retract Vol 1 (uL)") -> (decimal integer string=w3899:string)  [unwired: 1 in]
            n2682 = Concatenate Strings("tvolume  " ("string"), w3899, " u" ("string"), "\r") -> (w3896:string)
            n2683 = VISA Write(VISA resource name=w3897, write buffer=w3896) -> (VISA resource name out=w3893:refnum<visa-resource-name>)  [unwired: 1 in, 2 out]
            n2684 = Concatenate Strings("cvolume" ("string"), "\r") -> (w3894:string)
            n2685 = VISA Write(VISA resource name=w3893, write buffer=w3894) -> (VISA resource name out=w3888:refnum<visa-resource-name>)  [unwired: 1 in, 2 out]
            n2686 = Concatenate Strings("wrun" ("string"), "\r") -> (w3889:string)
            n2687 = VISA Write(VISA resource name=w3888, write buffer=w3889) -> ()  [unwired: 1 in, 3 out]
          }
        }
      }
      event "Flip Green Filter": Value Change {
        n2688 = event-data() -> ()  [unwired: 7 out]
        n2689 = Not(x="Flip Green Filter") -> (.not. x?=w3908:bool)
        n2690 = local write "Flip Green Filter"(w3908) -> ()
        n2691 = flat-sequence {
          tunnel: [w3917] -> w3913
          tunnel: [w3916] -> w3912
          tunnel: w3907 -> [w3915]
          tunnel: [w3920] -> w3911
          tunnel: w3913 -> [w3920]
          tunnel: [w3919] -> w3910
          tunnel: w3912 -> [w3919]
          tunnel: w3911 -> [w3924]
          tunnel: w3910 -> [w3923]
          tunnel: [w3922] -> w3914
          frame #0 {
            n2692 = xnode "Read/Write Control"("FPGA VI Reference In"=w3915, "Green Filter Flipper"=TRUE) -> ("FPGA VI Reference Out"=w3917:T25, "error out"=w3916:errorcluster)  [unwired: 1 in]
          }
          frame #1 {
            n2693 = Wait (ms)(milliseconds to wait=u32 100) -> ()  [unwired: 1 out]
          }
          frame #2 {
            n2694 = xnode "Read/Write Control"("FPGA VI Reference In"=w3924, "error in"=w3923, "Green Filter Flipper"=FALSE) -> ("error out"=w3922:errorcluster)  [unwired: 1 out]
          }
        }
      }
      event "Pump 1 contents", "Pump 3 contents": Value Change {
        n2695 = event-data() -> ()  [unwired: 7 out]
        n2696 = local read "Pump 1 contents"() -> (→"Pump 1 cont disp":string)
        n2697 = local read "Pump 3 contents"() -> (→"Pump 3 cont disp":string)
      }
      event "Reset Trap Pos. FB": Value Change {
        n2698 = event-data() -> ()  [unwired: 7 out]
        n2699 = xnode "Read/Write Control"("FPGA VI Reference In"=w3928, "Trap Pos. FB Reset"="Reset Trap Pos. FB") -> ()  [unwired: 1 in, 2 out]
      }
      event "Rem fb disp offset": Value Change {
        n2700 = event-data() -> ()  [unwired: 7 out]
        n2701 = local write "Rem fb disp offset"(FALSE ("Rem fb disp offset")) -> ()
        n2702 = local read "Mean T1 Position (nm)"() -> (w3931:dbl)
        n2703 = local read "FB Trap Pos Offset"() -> (w3932:dbl)
        n2704 = Subtract(x=w3932, y=w3931) -> (x-y=w3930:dbl)
        n2705 = local write "FB Trap Pos Offset"(w3930) -> ()
      }
      event "Threshold (nm)": Value Change {
        n2706 = event-data() -> ()  [unwired: 7 out]
        n2707 = flat-sequence {
          tunnel: [w3937] -> w3935
          tunnel: w3934 -> [w3936]
          tunnel: w3935 -> [w3948]
          frame #0 {
            n2708 = xnode "Read/Write Control"("FPGA VI Reference In"=w3936) -> ("FPGA VI Reference Out"=w3940:T25, "error out"=w3939:errorcluster, "FPGA TTrig Thresh"=w3941:i64)  [unwired: 1 in]
            n2709 = local read "Threshold stored (nm)"() -> (w3947:dbl)
            n2710 = local read "Threshold (nm)"() -> (w3937:dbl)
            n2711 = local read "AOM X Cal (nm/MHz)"() -> (w3945:dbl)
            n2712 = Subtract(x=w3937, y=w3947) -> (x-y=w3946:dbl)
            n2713 = Divide(x=w3946, y=w3945) -> (x/y=w3943:dbl)
            n2714 = call "IR AOM freq to word.vi"("Frequency In (MHz)"=w3943) -> ("Frequency Word Out (double)"=w3944:dbl)
            n2715 = To Quad Integer(1:w3944) -> (0:w3942:i64)
            n2716 = Add(x=w3941, y=w3942) -> (x+y=w3938:i64)
            n2717 = xnode "Read/Write Control"("FPGA VI Reference In"=w3940, "error in"=w3939, "FPGA TTrig Thresh"=w3938) -> ()  [unwired: 2 out]
          }
          frame #1 {
            "Threshold stored (nm)" <- w3948
          }
        }
      }
      event "FB Trig Integrate": Value Change {
        n2718 = event-data() -> ()  [unwired: 7 out]
        n2719 = local read "FB Trig Integrate"() -> (w3951:u32)
        n2720 = xnode "Read/Write Control"("FPGA VI Reference In"=w3949, "FB Trig Integrate"=w3951) -> ("error out"=w3950:errorcluster)  [unwired: 1 in, 1 out]
      }
      event "11": Value Change {
        n2721 = event-data() -> ()  [unwired: 7 out]
        n2722 = local read "11"() -> (w3952:bool)
        n2723 = case shown="True" w3952 {
          frame False {
          }
          frame True {
            n2724 = local read "Messages"() -> (w3954:string)
            n2725 = call "Update messages.vi"("Message to add"="You kicked it up to 11!", "Old message string"=w3954) -> ("New message string"=w3955:string)
            n2726 = call <vilib>:"Beep.vi"() -> ()  [unwired: 12 in]
            n2727 = local write "Messages"(w3955) -> ()
          }
        }
      }
      event "Trap Pos. FB ON": Value Change {
        n2728 = event-data() -> ()  [unwired: 7 out]
        n2729 = xnode "Read/Write Control"("FPGA VI Reference In"=w3956, "Force feedback"="Trap Pos. FB ON") -> ()  [unwired: 1 in, 2 out]
      }
      event "Remove Action Offset": Value Change {
        n2730 = event-data() -> ()  [unwired: 7 out]
        n2731 = local write "Remove Action Offset"(FALSE ("Remove Action Offset")) -> ()
        n2732 = local read "Trap Pos. FB Mult Factor"() -> (w3963:i64)
        n2733 = local read "Trap Pos FB Action"() -> (w3961:i64)
        n2734 = local read "Trap Pos. FB Offset Factor"() -> (w3959:i64)
        n2735 = Multiply(x=w3963, y=w3961) -> (x*y=w3962:i64)
        n2736 = Add(x=w3962, y=w3959) -> (x+y=w3960:i64)
        n2737 = local write "Trap Pos. FB Offset Factor"(w3960) -> ()
        n2738 = xnode "Read/Write Control"("FPGA VI Reference In"=w3958, "Trap Pos. FB Offset Factor"=w3960) -> ()  [unwired: 1 in, 2 out]
      }
      event "Remove Unwinding Offset": Value Change {
        n2739 = event-data() -> ()  [unwired: 7 out]
        n2740 = local write "Remove Unwinding Offset"(FALSE ("Remove Action Offset")) -> ()
        n2741 = local read "Trap Pos. FB Mult Factor"() -> (w3977:i64)
        n2742 = local read "Trap Pos FB Action"() -> (w3975:i64)
        n2743 = local read "Trap Pos. FB Offset Factor"() -> (w3974:i64)
        n2744 = Multiply(x=w3977, y=w3975) -> (x*y=w3976:i64)
        n2745 = local read "Trap Pos. FB Mult Factor"() -> (w3973:i64)
        n2746 = Add(x=w3976, y=w3974) -> (x+y=w3967:i64)
        n2747 = Multiply(x=32768, y="factor") -> (x*y=w3970:dbl)
        n2748 = Multiply(x=w3970, y=w3973) -> (x*y=w3972:dbl)
        n2749 = Subtract(x=w3967, y=w3972) -> (x-y=w3971:dbl)
        n2750 = To Quad Integer(1:w3971) -> (0:w3966:i64)
        n2751 = xnode "Read/Write Control"("FPGA VI Reference In"=w3965, "Trap Pos. FB Offset Factor"=w3966) -> ()  [unwired: 1 in, 2 out]
        n2752 = local write "Trap Pos. FB Offset Factor"(w3966) -> ()
      }
      event "Trap Pos. FB Range", "Trap Pos. FB Gains", "Trap Pos. FB Mult Factor", "Trap Pos. FB Offset Factor", "Trap Pos FB Negate Action", "Trap Pos FB Monitor\nT1 or T2", "Differential FB?", "Negate Diff?": Value Change {
        n2753 = event-data() -> ()  [unwired: 7 out]
        n2754 = Unbundle By Name("Trap Pos. FB Gains") -> ("proportional gain (Kc)"=w3982:fxp<+/-,16,8>, "integral gain (Kc*Ts/Ti)"=w3981:fxp<+/-,16,8>, "derivative gain (Kc*Td/Ts)"=w3980:fxp<+/-,16,8>)
        n2755 = local read "Negate Diff?"() -> (w3987:bool)
        n2756 = Unbundle By Name("Trap Pos. FB Range") -> ("output high"=w3985:fxp<+/-,16,1>, "output low"=w3984:fxp<+/-,16,1>)
        n2757 = xnode "Read/Write Control"("FPGA VI Reference In"=w3979, "FB2 output high"=w3985, "FB2 output low"=w3984, "P2"=w3982, "I2"=w3981, "D2"=w3980, "Trap Pos. FB Mult Factor"="Trap Pos. FB Mult Factor", "Trap Pos. FB Offset Factor"="Trap Pos. FB Offset Factor", "Trap Pos FB Negate Action"="Trap Pos FB Negate Action", "Trap Pos FB Monitor T1 or T2"="Trap Pos FB Monitor\nT1 or T2", "AI1 X Scale"="Trap Pos. AI1 X Pre-scale", "Negate Diff?"=w3987, "Diff FB Measurement?"="Differential FB?") -> ()  [unwired: 1 in, 2 out]
      }
      event "Trap Pos FB SP", "Trap Pos FB SP 2", "Use SP 2": Value Change {
        n2758 = event-data() -> ()  [unwired: 7 out]
        n2759 = Select(t="Trap Pos FB SP 2", s="Use SP 2", f="Trap Pos FB SP") -> (s? t:f=w3995:fxp<+/-,16,1>)
        n2760 = xnode "Read/Write Control"("FPGA VI Reference In"=w3994, "Trap Pos. FB SP"=w3995) -> ()  [unwired: 1 in, 2 out]
      }
      event "Offset SP2 from SP1": Value Change {
        n2761 = event-data() -> ()  [unwired: 7 out]
        n2762 = local read "Trap Pos FB SP"() -> (w4001:fxp<+/-,16,1>)
        n2763 = Add(x=w4001, y="SP2 Offset") -> (x+y=w3999:fxp<+/-,16,1>)
        n2764 = property on="Trap Pos FB SP 2" class="DigNum (strict)"("Val(Sgnl)"=w3999) -> ()  [unwired: 2 in, 2 out]
        n2765 = local write "Offset SP2 from SP1"(FALSE ("Offset SP2 from SP1")) -> ()
      }
      event "Set Reading to\nSetpoint": Value Change {
        # "This is the actual PID input signal"
        n2766 = event-data() -> ()  [unwired: 7 out]
        n2767 = local write "Set Reading to\nSetpoint"(FALSE ("Set SP to Reading")) -> ()
        n2768 = xnode "Read/Write Control"("FPGA VI Reference In"=w4003) -> ("FPGA VI Reference Out"=w4006:T25, "error out"=w4005:errorcluster, "Trap Pos FB Int-Norm Signal"=w4004:fxp<+/-,16,1>)  [unwired: 1 in]
        n2769 = local read "Differential FB?"() -> (w4007:bool)
